vi "PushLED.vi"(0 "Array":string[](array[string]), 5 "Strobe":refnum<vi>, 7 "Frequency":refnum<vi>, 9 "Duty":refnum<vi>, 11 "Voltage":refnum<vi>, 12 "StartTime":timestamp) -> (4 "Enqueue":string, 15 "Current Time":dbl)   [LabVIEW 2019, in "Scripts.lvclass"]
uses:
  Scripts.lvclass
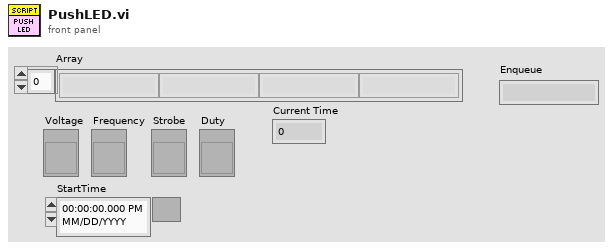
[diagram p1: front panel]
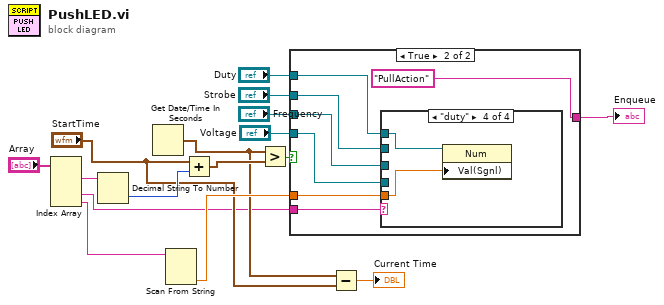
[diagram p0: block diagram]
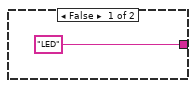
[diagram p2: hidden frame]
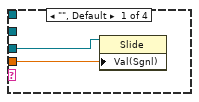
[diagram p3: hidden frame]
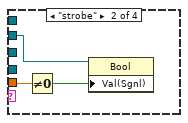
[diagram p4: hidden frame]
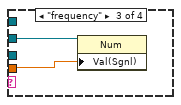
[diagram p5: hidden frame]
diagram:
  n1 = Index Array(array="Array") -> (element #1=w15:string, element #3=w4:string, element #4=w11:string)  [unwired: 4 in, 1 out]
  n2 = Decimal String To Number(string=w15) -> (number=w14:i32)  [unwired: 2 in, 1 out]
  n3 = Get Date/Time In Seconds() -> (seconds since 1Jan1904=w6:timestamp)
  n4 = Scan From String(input string=w11) -> (output 1=w9:dbl)  [unwired: 4 in, 3 out]
  n5 = Add(x="StartTime", y=w14) -> (x+y=w8:timestamp)
  n6 = Greater?(x=w6, y=w8) -> (0:w13:bool)
  n7 = case shown="True" w13 {
    tunnel: w9 -> [_ w24]
    tunnel: ["LED" ("element") "PullAction" ("element")] -> w12
    tunnel: "Voltage" -> [_ w22]
    tunnel: w4 -> [_ w21]
    tunnel: "Frequency" -> [_ w19]
    tunnel: "Strobe" -> [_ w20]
    tunnel: "Duty" -> [_ w18]
    frame False {
    }
    frame True {
      n8 = case shown="\"duty\"" w21 {
        tunnel: w24 -> [w26 w27 w30 w33]
        tunnel: w22 -> [w25 _ _ _]
        tunnel: w20 -> [_ w29 _ _]
        tunnel: w19 -> [_ _ w31 _]
        tunnel: w18 -> [_ _ _ w32]
        frame "", Default {
          n9 = property class="Slide"(reference=w25, "Val(Sgnl)"=w26) -> ()  [unwired: 1 in, 2 out]
        }
        frame "strobe" {
          n10 = Not Equal To 0?(x=w27) -> (x != 0?=w28:bool)
          n11 = property class="Bool"(reference=w29, "Val(Sgnl)"=w28) -> ()  [unwired: 1 in, 2 out]
        }
        frame "frequency" {
          n12 = property class="Num"(reference=w31, "Val(Sgnl)"=w30) -> ()  [unwired: 1 in, 2 out]
        }
        frame "duty" {
          n13 = property class="Num"(reference=w32, "Val(Sgnl)"=w33) -> ()  [unwired: 1 in, 2 out]
        }
      }
    }
  }
  "Enqueue" <- w12
  n14 = Subtract(x=w6, y="StartTime") -> (x-y=→"Current Time":dbl)
